vi "get unique file name.vi"(6 "size":i64, 7 "file directory":path, 8 "error in":errorcluster, 9 "file extension":string, 11 "file name":string) -> (0 "error out":errorcluster, 1 "Duplicate?":bool, 3 "unique file path":path)   [LabVIEW 2023, in "File Classes.lvlib"]
uses:
  File Classes.lvlib
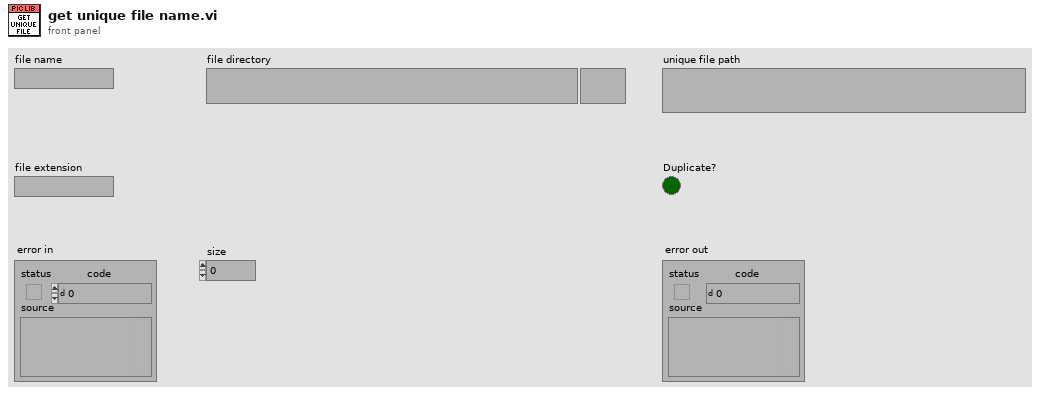
[diagram p1: front panel]
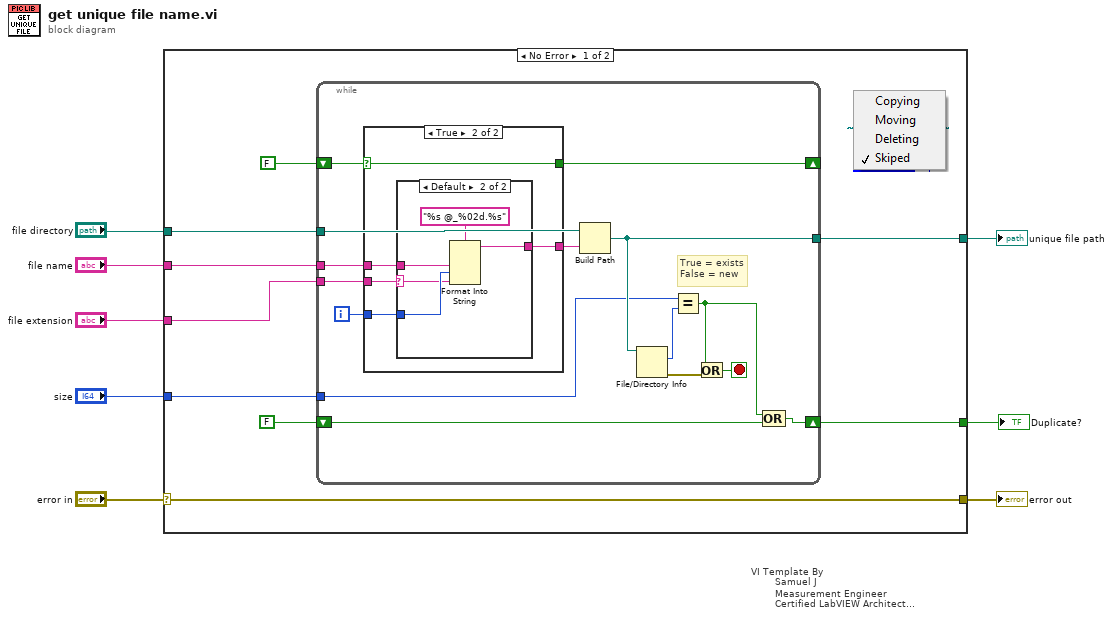
[diagram p0: block diagram]
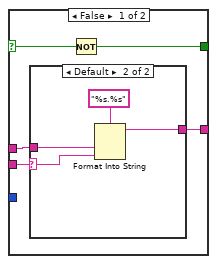
[diagram p2: hidden frame]
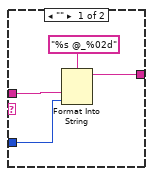
[diagram p4: hidden frame]
diagram:
  n1 = case "VI Template By\n        Samuel J\n        Measurement Engineer\n        Certified LabVIEW Architect\n        Vestas Technology R&D Chennai" shown="No Error" "error in" {
    selector: "error in" -> [w17 w58]
    tunnel: [w17 w58] -> w7
    tunnel: "file directory" -> [w13 w57]
    tunnel: [w15 w57] -> w5
    tunnel: [w9 _] -> w4
    tunnel: "size" -> [w14 _]
    tunnel: "file name" -> [w11 _]
    tunnel: "file extension" -> [w12 _]
    frame No Error {
      n2 = while {
        tunnel: w13 -> [w31]
        tunnel: w12 -> [w29]
        tunnel: [w28] -> w15
        shift-right: [w25] -> _
        shift-left: FALSE -> [w26]
        tunnel: w11 -> [w30]
        tunnel: w14 -> [w23]
        shift-right: [w21] -> w9
        shift-left: FALSE -> [w22]
        i -> [w24]
        stop <- w19 stop-if-true
        # "True = exists\nFalse = new"
        n3 = case shown="True" w26 {
          selector: w26 -> [w34 w45]
          tunnel: [w37 w47] -> w32
          tunnel: w30 -> [w36 w46]
          tunnel: w29 -> [w35 w43]
          tunnel: [w33 w45] -> w25
          tunnel: w24 -> [_ w44]
          frame False {
            n4 = case shown="Default" w35 {
              selector: w35 -> [_ w40]
              tunnel: [w38 w42] -> w37
              tunnel: w36 -> [w38 w41]
              frame "" {
              }
              frame Default {
                n5 = Format Into String(format string="%s.%s", w41, w40) -> (resulting string=w42:string)  [unwired: 2 in, 1 out]
              }
            }
            n6 = Not(x=w34) -> (.not. x?=w33:bool)
          }
          frame True {
            n7 = case shown="Default" w43 {
              selector: w43 -> [_ w52]
              tunnel: [w51 w56] -> w47
              tunnel: w46 -> [w50 w55]
              tunnel: w44 -> [w48 w53]
              frame "" {
                n8 = Format Into String(format string="%s @_%02d", w50, w48) -> (resulting string=w51:string)  [unwired: 2 in, 1 out]
              }
              frame Default {
                n9 = Format Into String(format string="%s @_%02d.%s", w55, w53, w52) -> (resulting string=w56:string)  [unwired: 2 in, 1 out]
              }
            }
          }
        }
        n10 = Build Path(base path=w31, name or relative path=w32) -> (appended path=w28:path)
        n11 = File/Directory Info(path=w28) -> (size=w27:i64, error out=w20:errorcluster)  [unwired: 1 in, 5 out]
        n12 = Equal?(x=w23, y=w27) -> (x = y?=w18:bool)
        n13 = Or(x=w18, y=w20) -> (x .or. y?=w19:bool)
        n14 = Compound Arithmetic op=OR(w18, w22) -> (w21:bool)
      }
    }
    frame Error {
    }
  }
  "error out" <- w7
  "unique file path" <- w5
  "Duplicate?" <- w4
